vi "Ini_file_read.vi"(0 "Config file path name":string="use default", 5 "Section Name":string="general", 7 "Key Name":string="test_pc_name", 11 "error in (no error)":errorcluster) -> (4 "Key data":string, 8 "KeyFound?":bool, 10 "Yes?":bool, 15 "error out":errorcluster)   [LabVIEW 2013]
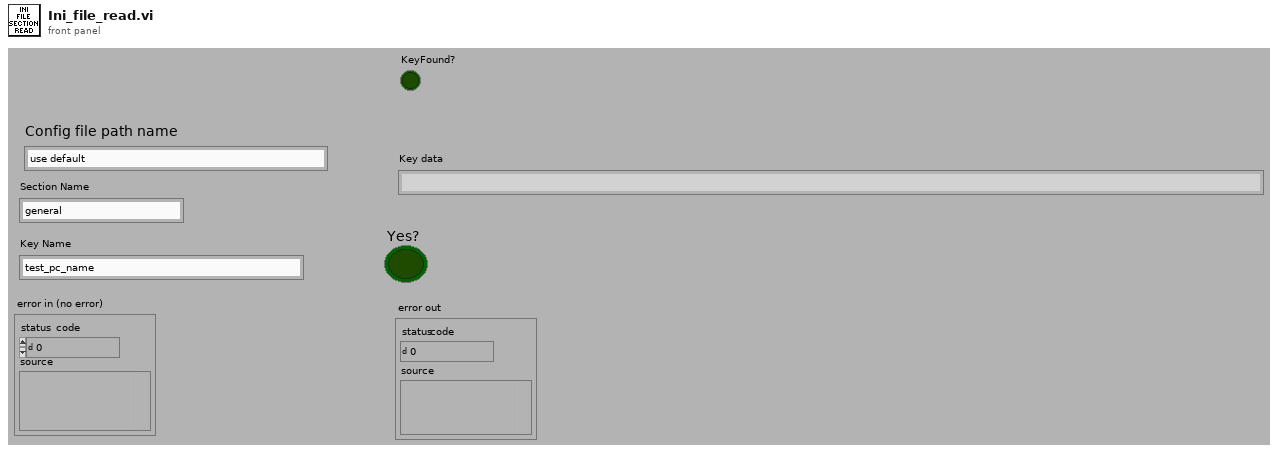
[diagram p1: front panel]
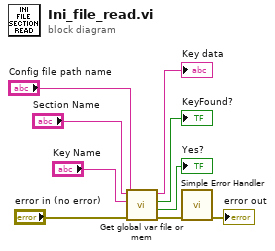
[diagram p0: block diagram]
diagram:
  n1 = call "Get global var file or mem.vi"("error in (no error)"="error in (no error)", "Config file path name"="Config file path name", "Key Name"="Key Name", "Section Name"="Section Name") -> ("error out"=w5:errorcluster, "Yes?"=→"Yes?":bool, "KeyFound?"=→"KeyFound?":bool, "Key data from file"=→"Key data":string)  [unwired: 4 in]
  n2 = call <vilib>:"Simple Error Handler.vi"("error in (no error)"=w5) -> ("error out"=→"error out":errorcluster)  [unwired: 4 in, 4 out]
